vi "Timer.vi"(0 "Wait_Time (10 s)":dbl=10.0 format="%#_13g", 11 "Error_In":errorcluster, 13 "Timer_Select":T1=enum."Time_Out?") -> (4 "Time_Out?":bool, 15 "Error_Out":errorcluster)   [LabVIEW 2023]
doc: "Used for time out opertion."
uses:
  Controls/Timer_Select.ctl
  Controls/Timer_Data.ctl
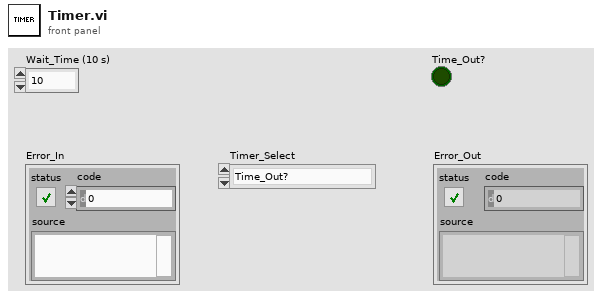
[diagram p1: front panel]
types:
  T1 = typedef "Timer_Select.ctl" = enum16{"Start_Timer", "Time_Out?", "Stop_Timer"}
  T2 = typedef "Timer_Data.ctl" = cluster{"Start_Time":dbl, "Start?":bool, "Wait_Time":dbl}
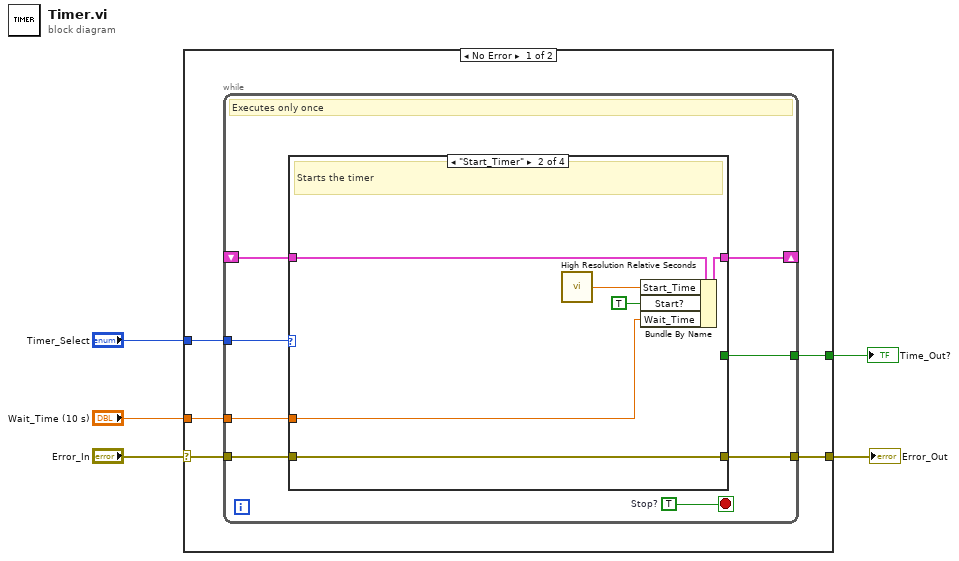
[diagram p0: block diagram]
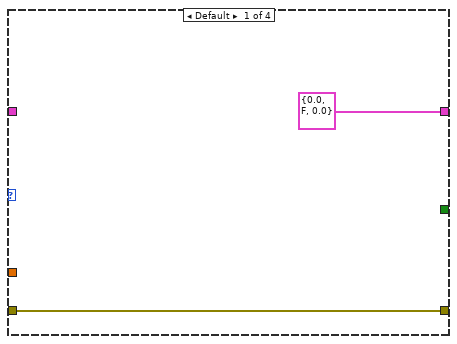
[diagram p2: hidden frame]
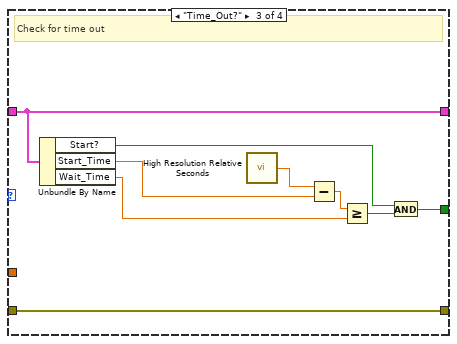
[diagram p3: hidden frame]
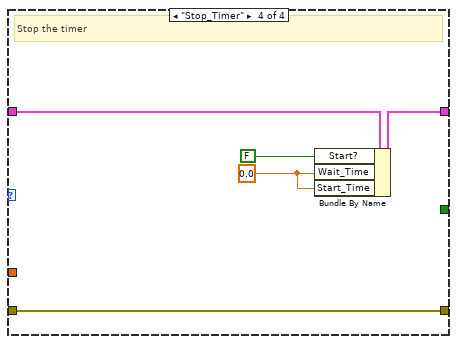
[diagram p4: hidden frame]
diagram:
  n1 = case shown="No Error" "Error_In" {
    selector: "Error_In" -> [w6 w41]
    tunnel: [w10 _] -> w5
    tunnel: [w9 w41] -> w4
    tunnel: "Wait_Time (10 s)" -> [w8 _]
    tunnel: "Timer_Select" -> [w7 _]
    frame No Error {
      n2 = while {
        tunnel: w7 -> [w18]
        shift-right: [w17] -> _
        shift-left: _ -> [w16]
        tunnel: [w15] -> w10
        tunnel: w6 -> [w13]
        tunnel: [w12] -> w9
        tunnel: w8 -> [w11]
        stop <- w14 stop-if-true
        w14 = TRUE  # Stop?
        # "Executes only once"
        n3 = case shown="\"Start_Timer\"" w18 {
          tunnel: [T2 {"Start_Time"=0.0, "Start?"=FALSE, "Wait_Time"=0.0} ("Cluster") w24 w30 w38] -> w17
          tunnel: w16 -> [_ w25 w30 w39]
          tunnel: [_ _ w31 _] -> w15
          tunnel: w13 -> [w20 w26 w33 w40]
          tunnel: [w20 w26 w33 w40] -> w12
          tunnel: w11 -> [_ w21 _ _]
          frame Default {
          }
          frame "Start_Timer" {
            # "Starts the timer"
            n4 = call <vilib>:"High Resolution Relative Seconds.vi"() -> ("relative seconds"=w23:dbl)
            n5 = Bundle By Name(cluster=w25, "Start_Time"=w23, "Start?"=TRUE, "Wait_Time"=w21) -> (w24:T2)
          }
          frame "Time_Out?" {
            # "Check for time out"
            n6 = Unbundle By Name(w30) -> ("Start?"=w28:bool, "Start_Time"=w29:dbl, "Wait_Time"=w27:dbl)
            n7 = call <vilib>:"High Resolution Relative Seconds.vi"() -> ("relative seconds"=w32:dbl)
            n8 = Subtract(x=w32, y=w29) -> (x-y=w35:dbl)
            n9 = Greater Or Equal?(x=w35, y=w27) -> (x >= y?=w34:bool)
            n10 = And(x=w28, y=w34) -> (x .and. y?=w31:bool)
          }
          frame "Stop_Timer" {
            w36 = 0.0 ("Wait_Time")
            # "Stop the timer"
            n11 = Bundle By Name(cluster=w39, "Start?"=FALSE, "Wait_Time"=w36, "Start_Time"=w36) -> (w38:T2)
          }
        }
      }
    }
    frame Error {
    }
  }
  "Time_Out?" <- w5
  "Error_Out" <- w4
